vi "Init.vi"(8 "error in (no error)":errorcluster, 9 "Reset (True)":bool=TRUE, 10 "Serial Configuration":T1={"Baud Rate"=9600, "Parity"=0, "Data Bits"=8, "Stop Bits"=10, "Flow Control"=0} {"Flow Control" items=["None", "XON/XOFF", "RTS/CTS", "XON/XOFF & RTS/CTS", "DTR/DSR", "XON/XOFF & DTR/DSR"]; "Stop Bits" items=["1.0"=10, "1.5"=15, "2.0"=20]; "Data Bits" items=["7"=7, "8"=8]; "Parity" items=["None", "Odd", "Even", "Mark", "Space"]; "Baud Rate" items=["300"=300, "600"=600, "1200"=1200, "2400"=2400, "4800"=4800, "9600"=9600, "19200"=19200]}, 11 "VISA resource name":refnum<visa-resource-name>) -> (0 "error out":errorcluster, 3 "VISA resource out":refnum<visa-resource-name>)   [LabVIEW 2017]
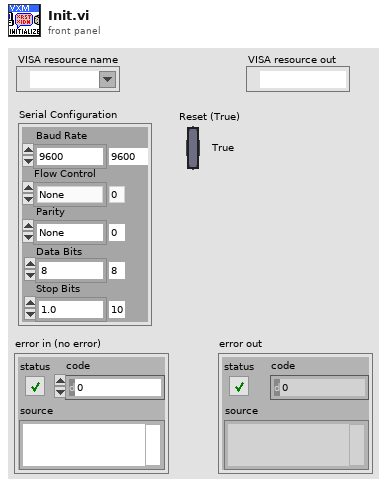
[diagram p1: front panel]
types:
  T1 = cluster{"Baud Rate":u32, "Parity":u16, "Data Bits":u16, "Stop Bits":u16, "Flow Control":u16}
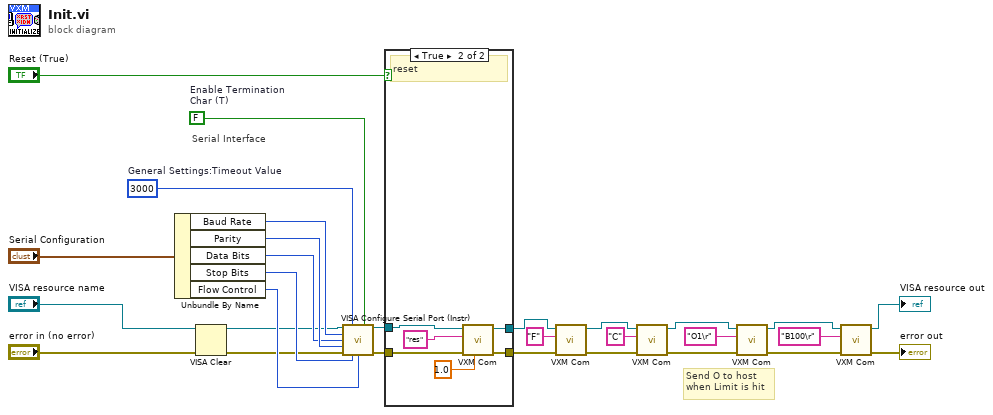
[diagram p0: block diagram]
diagram:
  w19 = FALSE  # Enable Termination Char (T)
  w20 = u32 3000  # General Settings:Timeout Value
  # "Send O to host\nwhen Limit is hit"
  # "Serial Interface"
  n1 = Unbundle By Name("Serial Configuration") -> ("Baud Rate"=w24:u32, "Parity"=w26:u16, "Data Bits"=w25:u16, "Stop Bits"=w27:u16, "Flow Control"=w28:u16)
  n2 = VISA Clear(VISA resource name="VISA resource name", error in (no error)="error in (no error)") -> (VISA resource name out=w22:refnum<visa-resource-name>, error out=w23:errorcluster)
  n3 = call <vilib>:"VISA Configure Serial Port (Instr).vi"("VISA resource name"=w22, "timeout (10sec)"=w20, "Enable Termination\nChar (T)"=w19, "baud rate (9600)"=w24, "data bits (8)"=w25, "parity (0:none)"=w26, "error in (no error)"=w23, "stop bits (10: 1 bit)"=w27, "flow control (0:none)"=w28) -> ("VISA resource name out"=w17:refnum<visa-resource-name>, "error out"=w16:errorcluster)  [unwired: 5 in]
  n4 = case shown="True" "Reset (True)" {
    tunnel: w17 -> [w30 w36]
    tunnel: w16 -> [w29 w35]
    tunnel: [w30 w32] -> w11
    tunnel: [w29 w31] -> w13
    frame False {
    }
    frame True {
      # "reset"
      n5 = call "VXM Com.vi"("Timeout, s"=1.0, "error in (no error)"=w35, "Write Buffer ('/' codes)"="res" ("Write Buffer"), "VISA resource name"=w36) -> ("error out"=w31:errorcluster, "VISA resource out"=w32:refnum<visa-resource-name>)  [unwired: 5 in, 1 out]
    }
  }
  n6 = call "VXM Com.vi"("error in (no error)"=w13, "Write Buffer ('/' codes)"="F" ("Write Buffer"), "VISA resource name"=w11) -> ("error out"=w9:errorcluster, "VISA resource out"=w8:refnum<visa-resource-name>)  [unwired: 6 in, 1 out]
  n7 = call "VXM Com.vi"("error in (no error)"=w9, "Write Buffer ('/' codes)"="C" ("Write Buffer"), "VISA resource name"=w8) -> ("error out"=w6:errorcluster, "VISA resource out"=w5:refnum<visa-resource-name>)  [unwired: 6 in, 1 out]
  n8 = call "VXM Com.vi"("error in (no error)"=w6, "Write Buffer ('/' codes)"="O1\r" ("Write Buffer"), "VISA resource name"=w5) -> ("error out"=w2:errorcluster, "VISA resource out"=w3:refnum<visa-resource-name>)  [unwired: 6 in, 1 out]
  "VISA resource out" <- w3
  n9 = call "VXM Com.vi"("error in (no error)"=w2, "Write Buffer ('/' codes)"="B100\r" ("Write Buffer"), "VISA resource name"=w3) -> ("error out"=→"error out":errorcluster)  [unwired: 6 in, 2 out]
